vi "CreatePizza.vi"(8 "error in (no error)":errorcluster, 10 "Pizza to order":T1, 11 "ChicagoPizzaStore in":refnum<class "ChicagoPizzaStore.lvclass">) -> (0 "error out":errorcluster, 2 "Pizza object":refnum<class "Pizza.lvclass">, 3 "ChicagoPizzaStore out":refnum<class "ChicagoPizzaStore.lvclass">)   [LabVIEW 2021, in "ChicagoPizzaStore.lvclass"]
uses:
  ChicagoPizzaStore.lvclass
  Pizza/pizza types.ctl
  Pizza/Pizza.lvclass
  ChicagoStyleCheesePizza/ChicagoStyleCheesePizza.lvclass
  C:/Users/nina/Documents/Head First Design Patterns/HeadFirstDesignPatternsLabVIEWandPython/04 Factory/LabVIEW/Pizza/Pizza.lvclass
  ChicagoStylePepeproniPizza/ChicagoStylePepperoniPizza.lvclass
panel:
  # "Connector Pane"
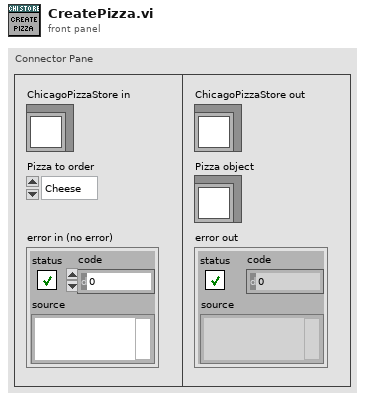
[diagram p1: front panel]
types:
  T1 = typedef "Pizza.lvclass/pizza types.ctl" = enum16{"Cheese", "Pepperoni"}
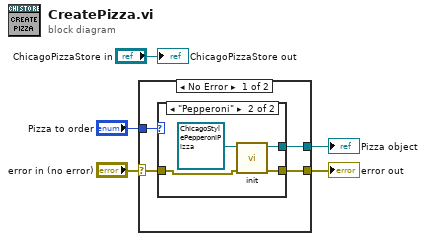
[diagram p0: block diagram]
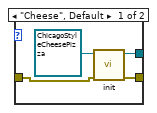
[diagram p2: hidden frame]
diagram:
  n1 = case shown="No Error" "error in (no error)" {
    selector: "error in (no error)" -> [w7 w18]
    tunnel: "Pizza to order" -> [w9 _]
    tunnel: [w8 _] -> w4
    tunnel: [w6 w18] -> w1
    frame No Error {
      n2 = case shown="\"Pepperoni\"" w9 {
        tunnel: [w12 w16] -> w8
        tunnel: w7 -> [w11 w15]
        tunnel: [w10 w14] -> w6
        frame "Cheese", Default {
          n3 = call "init.vi"("error in (no error)"=w11, "ChicagoStyleCheesePizza in"=refnum<class "ChicagoStyleCheesePizza.lvclass"> refnum ("ChicagoStyleCheesePizza.lvclass")) -> ("error out"=w10:errorcluster, "ChicagoStyleCheesePizza out"=w12:refnum<class "ChicagoStyleCheesePizza.lvclass">)  [unwired: 8 in]
        }
        frame "Pepperoni" {
          n4 = call "init.vi"("error in (no error)"=w15, "NYStyleCheesePizza in"=refnum<class "ChicagoStylePepperoniPizza.lvclass"> refnum ("ChicagoStylePepperoniPizza.lvclass")) -> ("error out"=w14:errorcluster, "NYStyleCheesePizza out"=w16:refnum<class "ChicagoStylePepperoniPizza.lvclass">)  [unwired: 8 in]
        }
      }
    }
    frame Error {
    }
  }
  "error out" <- w1
  "Pizza object" <- w4
  "ChicagoPizzaStore out" <- "ChicagoPizzaStore in"
